vi "DDMs_low_initialize_backup.vi"(7 "Measurement":T1(ring), 8 "error in (no error)":errorcluster, 10 "Device":enum16{"Agilent34401A", "ADCMT7351", "HP3478A"}(ring), 11 "VISA resource name":refnum<visa-resource-name>) -> (0 "error out":errorcluster, 3 "VISA resource name out":refnum<visa-resource-name>)   [LabVIEW 2017]
uses:
  <instrlib>/Agilent 34401/Agilent 34401.lvlib
  istr.lib/ADCMT7351_ADC/ADCMT7351_ADC.lvlib
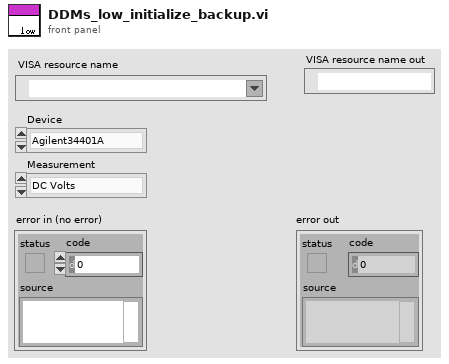
[diagram p1: front panel]
types:
  T1 = enum16{"DC Volts", "DC Currents", "2-Wire Resistance", "4-Wire Resistance"}
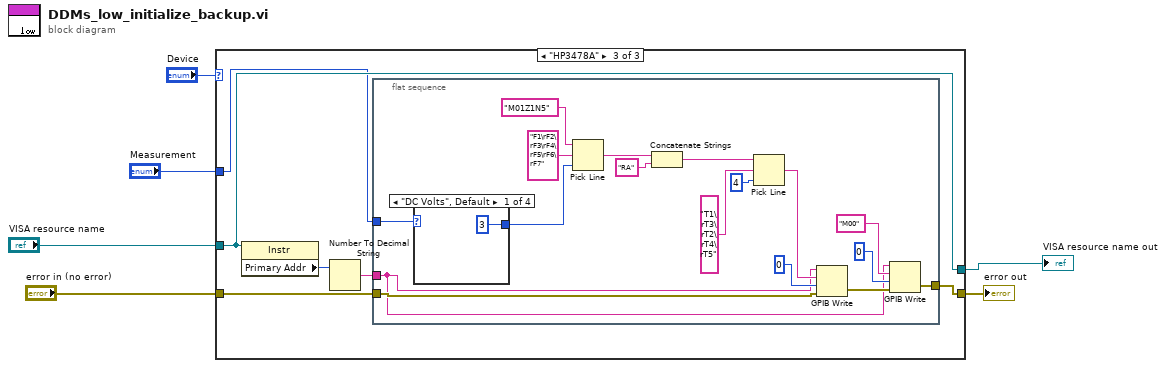
[diagram p0: block diagram]
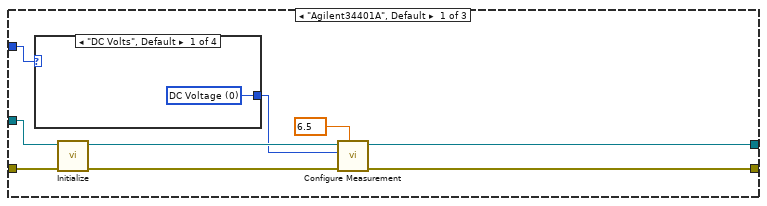
[diagram p2: hidden frame]
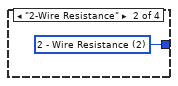
[diagram p3: hidden frame]
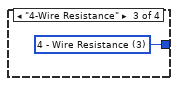
[diagram p4: hidden frame]
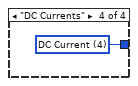
[diagram p5: hidden frame]
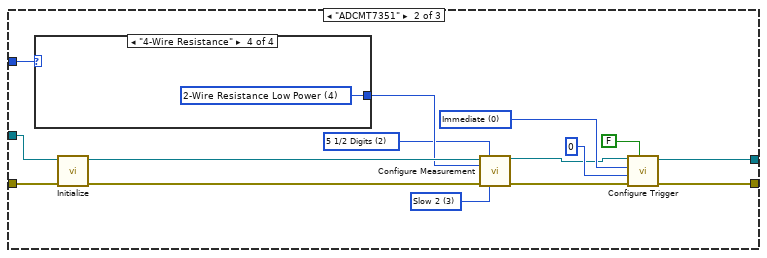
[diagram p6: hidden frame]
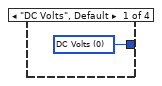
[diagram p7: hidden frame]
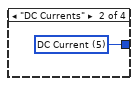
[diagram p8: hidden frame]
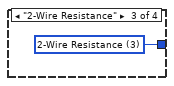
[diagram p9: hidden frame]
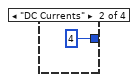
[diagram p10: hidden frame]
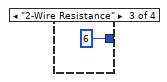
[diagram p11: hidden frame]
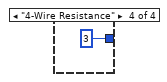
[diagram p12: hidden frame]
diagram:
  n1 = case shown="\"HP3478A\"" "Device" {
    tunnel: "VISA resource name" -> [w15 w34 w44]
    tunnel: "error in (no error)" -> [w14 w33 w40]
    tunnel: "Measurement" -> [w13 w30 w42]
    tunnel: [w8 w21 w44] -> w2
    tunnel: [w7 w23 w39] -> w1
    frame "Agilent34401A", Default {
      w9 = 6.5 items=["4.5"=4.5, "5.5"=5.5, "6.5"=6.5] ("Manual Resolution (5.5 Digits)")
      n2 = case shown="\"DC Volts\", Default" w13 {
        tunnel: [w16 w17 w18 w19] -> w10
        frame "DC Volts", Default {
          w16 = u16 0 items=["DC Voltage", "AC Voltage", "2 - Wire Resistance", "4 - Wire Resistance", "DC Current", "AC Current", "Frequency", "Period", "Continuity", "Diode Checking", "VDC:VDC Ratio", "Temperature", "Capacitance"] ("Function (0: DC Voltage)")
        }
        frame "2-Wire Resistance" {
          w17 = u16 2 items=["DC Voltage", "AC Voltage", "2 - Wire Resistance", "4 - Wire Resistance", "DC Current", "AC Current", "Frequency", "Period", "Continuity", "Diode Checking", "VDC:VDC Ratio", "Temperature", "Capacitance"] ("Function (0: DC Voltage)")
        }
        frame "4-Wire Resistance" {
          w18 = u16 3 items=["DC Voltage", "AC Voltage", "2 - Wire Resistance", "4 - Wire Resistance", "DC Current", "AC Current", "Frequency", "Period", "Continuity", "Diode Checking", "VDC:VDC Ratio", "Temperature", "Capacitance"] ("Function (0: DC Voltage)")
        }
        frame "DC Currents" {
          w19 = u16 4 items=["DC Voltage", "AC Voltage", "2 - Wire Resistance", "4 - Wire Resistance", "DC Current", "AC Current", "Frequency", "Period", "Continuity", "Diode Checking", "VDC:VDC Ratio", "Temperature", "Capacitance"] ("Function (0: DC Voltage)")
        }
      }
      n3 = call <instrlib>:"Initialize.vi"("error in (no error)"=w14, "VISA resource name"=w15) -> ("error out"=w11:errorcluster, "VISA resource name out"=w12:refnum<visa-resource-name>)  [unwired: 8 in]
      n4 = call <instrlib>:"Configure Measurement.vi"("Manual Resolution (5.5 Digits)"=w9, "error in (no error)"=w11, "Function (0: DC Voltage)"=w10, "VISA resource name"=w12) -> ("error out"=w7:errorcluster, "VISA resource name out"=w8:refnum<visa-resource-name>)  [unwired: 6 in]
    }
    frame "ADCMT7351" {
      w26 = u16 0 items=["Immediate", "Manual", "External", "Bus"] ("Trigger Source")
      w27 = u16 3 items=["Fast", "Medium", "Slow 1", "Slow 2"] ("Sampling Rate (3: Slow 2)")
      w28 = u16 2 items=["3 1/2 Digits", "4 1/2 Digits", "5 1/2 Digits"] ("Digits (2: 5 1/2)")
      n5 = case shown="\"4-Wire Resistance\"" w30 {
        tunnel: [w35 w36 w37 w38] -> w29
        frame "DC Volts", Default {
          w35 = u16 0 items=["DC Volts", "AC Volts", "AC+DC Volts", "2-Wire Resistance", "2-Wire Resistance Low Power", "DC Current", "AC Current", "AC+DC Current", "Diode", "Continuity", "Frequency"] ("Function (0: DC Volts)")
        }
        frame "DC Currents" {
          w36 = u16 5 items=["DC Volts", "AC Volts", "AC+DC Volts", "2-Wire Resistance", "2-Wire Resistance Low Power", "DC Current", "AC Current", "AC+DC Current", "Diode", "Continuity", "Frequency"] ("Function (0: DC Volts)")
        }
        frame "2-Wire Resistance" {
          w37 = u16 3 items=["DC Volts", "AC Volts", "AC+DC Volts", "2-Wire Resistance", "2-Wire Resistance Low Power", "DC Current", "AC Current", "AC+DC Current", "Diode", "Continuity", "Frequency"] ("Function (0: DC Volts)")
        }
        frame "4-Wire Resistance" {
          w38 = u16 4 items=["DC Volts", "AC Volts", "AC+DC Volts", "2-Wire Resistance", "2-Wire Resistance Low Power", "DC Current", "AC Current", "AC+DC Current", "Diode", "Continuity", "Frequency"] ("Function (0: DC Volts)")
        }
      }
      n6 = call <instrlib>:"Initialize.vi"("error in (no error)"=w33, "VISA resource name"=w34) -> ("error out"=w31:errorcluster, "VISA resource name out"=w32:refnum<visa-resource-name>)  [unwired: 8 in]
      n7 = call <instrlib>:"Configure Measurement.vi"("VISA resource name"=w32, "Digits (2: 5 1/2)"=w28, "Function (0: DC Volts)"=w29, "error in (no error)"=w31, "Sampling Rate (3: Slow 2)"=w27) -> ("VISA resource name out"=w22:refnum<visa-resource-name>, "error out"=w24:errorcluster)  [unwired: 9 in]
      n8 = call "Configure Trigger.vi"("Enable Trigger Delay (Enable)"=FALSE, "error in (no error)"=w24, "Trigger Delay (0 second)"=0, "Trigger Source (0: Immediate)"=w26, "VISA resource name"=w22) -> ("error out"=w23:errorcluster, "VISA resource name out"=w21:refnum<visa-resource-name>)  [unwired: 5 in]
    }
    frame "HP3478A" {
      n9 = property class="Instr"(reference=w44) -> ("Primary Addr"=w43:u16)  [unwired: 1 in, 2 out]
      n10 = Number To Decimal String(number=w43) -> (decimal integer string=w41:string)  [unwired: 1 in]
      n11 = flat-sequence {
        tunnel: w42 -> [w56]
        tunnel: w41 -> [w45]
        tunnel: w40 -> [w50]
        tunnel: [w46] -> w39
        frame #0 {
          n12 = case shown="\"DC Volts\", Default" w56 {
            tunnel: [3 ("line index") 4 ("line index") 6 ("line index") 3 ("line index")] -> w55
            frame "DC Volts", Default {
            }
            frame "DC Currents" {
            }
            frame "2-Wire Resistance" {
            }
            frame "4-Wire Resistance" {
            }
          }
          n13 = Pick Line(string ("")="M01Z1N5", multi-line string="F1\rF2\rF3\rF4\rF5\rF6\rF7", line index=w55) -> (output string=w54:string)
          n14 = Concatenate Strings(w54, "RA") -> (w52:string)
          n15 = Pick Line(string ("")=w52, multi-line string="T1\rT3\rT2\rT4\rT5", line index=4) -> (output string=w61:string)
          n16 = GPIB Write(0:w45, 1:w61, 2:0, 3:w50) -> (6:w47:errorcluster)  [unwired: 1 in, 1 out]
          n17 = GPIB Write(0:w45, 1:"M00", 2:0, 3:w47) -> (6:w46:errorcluster)  [unwired: 1 in, 1 out]
        }
      }
    }
  }
  "VISA resource name out" <- w2
  "error out" <- w1
